vi "GeolocationEnergySNRvariationTxswitching.vi"() -> ()   [LabVIEW 2012]
uses:
  <vilib>/addons/database/Connection.llb/DB Tools Open Connec (Path).vi
  <vilib>/measure/maspectr.llb/FFT Power Spectrum and PSD for 1 Chan.vi
  <instrlib>/niUSRP/niUSRP Fetch Rx Data (CDB Cluster).vi
  <vilib>/addons/Modulation/Digital/General/MT Generate PSK System Parameters(M).vi
  <instrlib>/niUSRP/niUSRP Write Tx Data (CDB Cluster).vi
  <vilib>/addons/Modulation/niDMT.lvlib
  <vilib>/measure/NI_MAPro.lvlib
  <vilib>/addons/database/NI_Database_API.lvlib
panel:
  out "Power Spectrum / PSD":cluster{"f0":dbl, "df":dbl, "magnitude":dbl[]} {"magnitude" format="%.2p"; "f0" format="%0.2p"; "df" format="%0.2p"}
  out "SNR":dbl
  out "x/y":dbl
  in  "IQ rate":dbl=100000.0 format="%#_6p"
  in  "gain":dbl format="%#_6f"
  out "Channel is free":bool
  in  "Boolean":bool
  out "data":variant[][](array[variant])
  out "columns":string[](array[string])
  in  "connection information":path
  out "product":i32
  out "output array":variant[](array[variant])
  out "cluster":T1
  out "data 2":dbl
  out "String":string
  out "millisecond timer value":u32
  out "Entering into 2nd \n          Loop":string
  out "Symbol Rate\n[symbols/sec]":dbl=25000.0 format="%#.6p"
  in  "BPSK System Parameters 9":T2={"Samples per Symbol"=8, "symbol map"=[], "Differential PSK"=enum."disable", "PSK type"=0} caption="BPSK System Parameters" {"PSK type" items=["normal", "shifted", "offset"]; "symbol map" format="%.3f"}
  in  "BPSK System Parameters 8":T2={"Samples per Symbol"=8, "symbol map"=[], "Differential PSK"=enum."disable", "PSK type"=0} caption="BPSK System Parameters" {"PSK type" items=["normal", "shifted", "offset"]; "symbol map" format="%.3f"}
  in  "BPSK System Parameters 7":T2={"Samples per Symbol"=8, "symbol map"=[], "Differential PSK"=enum."disable", "PSK type"=0} caption="BPSK System Parameters" {"PSK type" items=["normal", "shifted", "offset"]; "symbol map" format="%.3f"}
  in  "BPSK System Parameters 6":T2={"Samples per Symbol"=8, "symbol map"=[], "Differential PSK"=enum."disable", "PSK type"=0} caption="BPSK System Parameters" {"PSK type" items=["normal", "shifted", "offset"]; "symbol map" format="%.3f"}
  in  "BPSK System Parameters 5":T2={"Samples per Symbol"=8, "symbol map"=[], "Differential PSK"=enum."disable", "PSK type"=0} caption="BPSK System Parameters" {"PSK type" items=["normal", "shifted", "offset"]; "symbol map" format="%.3f"}
  in  "BPSK System Parameters 4":T2={"Samples per Symbol"=8, "symbol map"=[], "Differential PSK"=enum."disable", "PSK type"=0} caption="BPSK System Parameters" {"PSK type" items=["normal", "shifted", "offset"]; "symbol map" format="%.3f"}
  in  "BPSK System Parameters 3":T2={"Samples per Symbol"=8, "symbol map"=[], "Differential PSK"=enum."disable", "PSK type"=0} caption="BPSK System Parameters" {"PSK type" items=["normal", "shifted", "offset"]; "symbol map" format="%.3f"}
  in  "Tab Control":T3(tab)
  in  "Enter control signal (1,2 or 3)":string
  in  "Packet Parameters":T4={"Guard Bits "=30, "Sync Bits"=20, "Message Bits"=128}
  in  "Packet Pad \n[samples]":i32=200
  in  "Blank Frame \n[samples]":i32=500
  out "Number of Packets in Message":i32=46
  in  "PN sequence order\nfor Sync Bits":i32=31 caption="PN sequence order (9)"
  in  "Packet Repeat":i32=2
  in  "Pulse Shaping Filter Parameters":T5={"Alpha"=0.5, "Filter Length"=6, "TX Filter"=enum."Root Raised Cos"} caption="Pulse Shaping Filter" {"Alpha" format="%.2f"}
  out "Actual Tx Parameters":T6={"Tx IQ Sampling\nRate [s/sec]"=200000.0, "Tx Frequency [Hz]"=2500000000.0, "Tx Gain [dB]"=0.0, "Tx Antenna"="TX1"} {"Tx Gain [dB]" format="%#.6p"; "Tx Frequency [Hz]" format="%#.6p"; "Tx IQ Sampling\nRate [s/sec]" format="%#.6p"}
  in  "USRP IP address":refnum<k15>="192.168.10.2"
  out "error out":errorcluster
  in  "Queue Length":i32=10
  out "Transmission\n       Stop":bool
  in  "end of data?":bool
  out "Constellation Graph":T7(graph)
  in  "autoscale":bool
  out "millisecond timer value 2":u32
  out "x = y?":bool
  out "Transmission\n      Time":bool
  out "error out 2":errorcluster
  out "Message Text 3":string="Two roads diverged in a yellow wood,\nAnd sorry I could not travel both\nAnd be one traveler, long I stood\nAnd looked down one as far as I could\nTo where it bent in the undergrowth.\n\nThen took the other, as just as fair,\nAnd having perhaps the better claim,\nBecause it was grassy and wanted wear;\nThough as for that the passing there\nHad worn them really about the same.\n\nAnd both that morning equally lay\nIn leaves no step had trodden black.\nOh, I kept the first for another day!\nYet knowing how way leads on to way,\nI doubted if I should ever come back.\n\nI shall be telling this with a sigh\nSomewhere ages and ages hence:\nTwo roads diverged in a wood, and I--\nI took the one less traveled by,\nAnd that has made all the difference.\n"
  out "M-PSK (4)":i32
  out "Required Power":dbl
  in  "Referance Cluster":T6={"Tx IQ Sampling\nRate [s/sec]"=500000.0, "Tx Frequency [Hz]"=2500000000.0, "Tx Gain [dB]"=0.0, "Tx Antenna"="TX1"} {"Tx Gain [dB]" format="%#.6p"; "Tx Frequency [Hz]" format="%#.6p"; "Tx IQ Sampling\nRate [s/sec]" format="%#.6p"}
  out "output cluster":T6
  out "Numeric":u32
  # "Guard\nBand"
  # "Sync\nSeq"
  # "Packet\nNumber"
  # "Pad\nData"
  # "Blank\nFrame"
  # "Data"
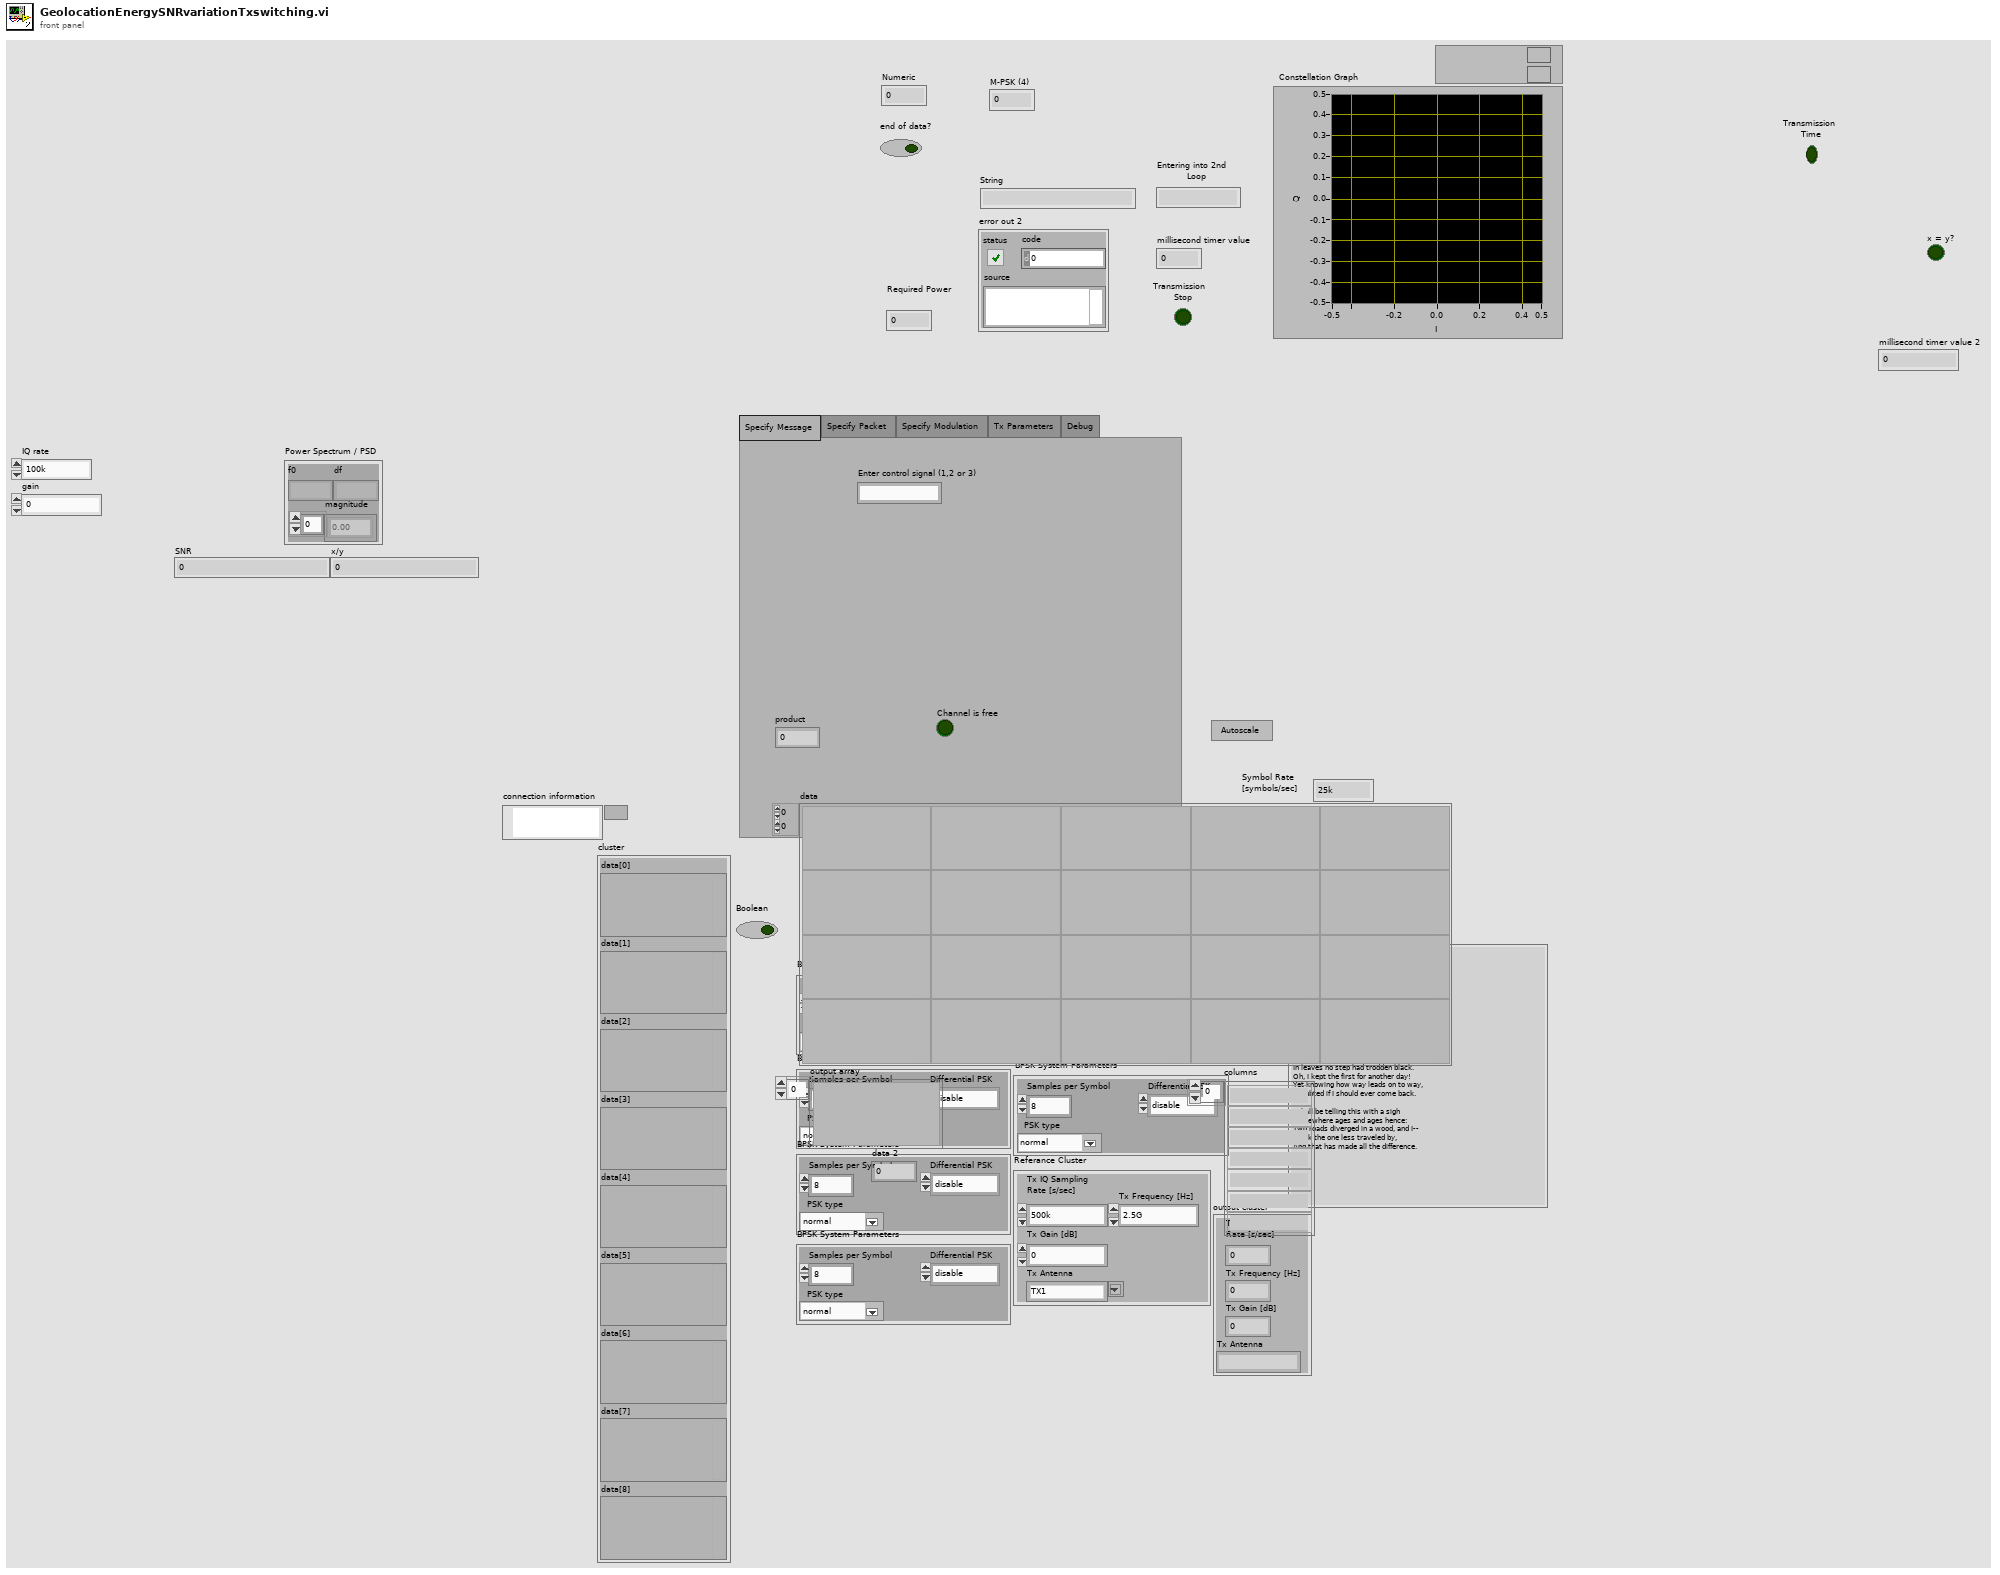
[diagram p1: front panel]
types:
  T1 = cluster{"data[0]":variant, "data[1]":variant, "data[2]":variant, "data[3]":variant, "data[4]":variant, "data[5]":variant, "data[6]":variant, "data[7]":variant, "data[8]":variant}
  T2 = cluster{"Samples per Symbol":i32, "symbol map":cdb[], "Differential PSK":enum16{"disable", "enable"}, "PSK type":u16}
  T3 = enum32{"Specify Message", "Specify Packet", "Specify Modulation", "Tx Parameters", "Debug"}
  T4 = cluster{"Guard Bits ":i32, "Sync Bits":i32, "Message Bits":i32}
  T5 = cluster{"Alpha":dbl, "Filter Length":i32, "TX Filter":enum16{"none", "Raised Cosine", "Root Raised Cos", "Gaussian"}}
  T6 = cluster{"Tx IQ Sampling\nRate [s/sec]":dbl, "Tx Frequency [Hz]":dbl, "Tx Gain [dB]":dbl, "Tx Antenna":string}
  T7 = cluster{"Decimated Array":dbl[], "Decimated Array":dbl[]}[]
  T8 = typedef "NI_Database_API.lvlib/Conn ObjectReference.ctl" = refnum<k1>
  T9 = cluster{"samples per symbol (16)":i32, "symbol map":cdb[], "differential PSK":enum16{"disable", "enable"}, "PSK type":u16}
  T10 = cluster{"s? t:f":cluster{"t0":dbl, "dt":dbl, "Y":cdb[]}, i32}
  T11 = cluster{"output complex waveform":cluster{"t0":dbl, "dt":dbl, "Y":cdb[]}, i32}
  T12 = cluster{"constellation":dbl[], "oversampled data":dbl[]}[]
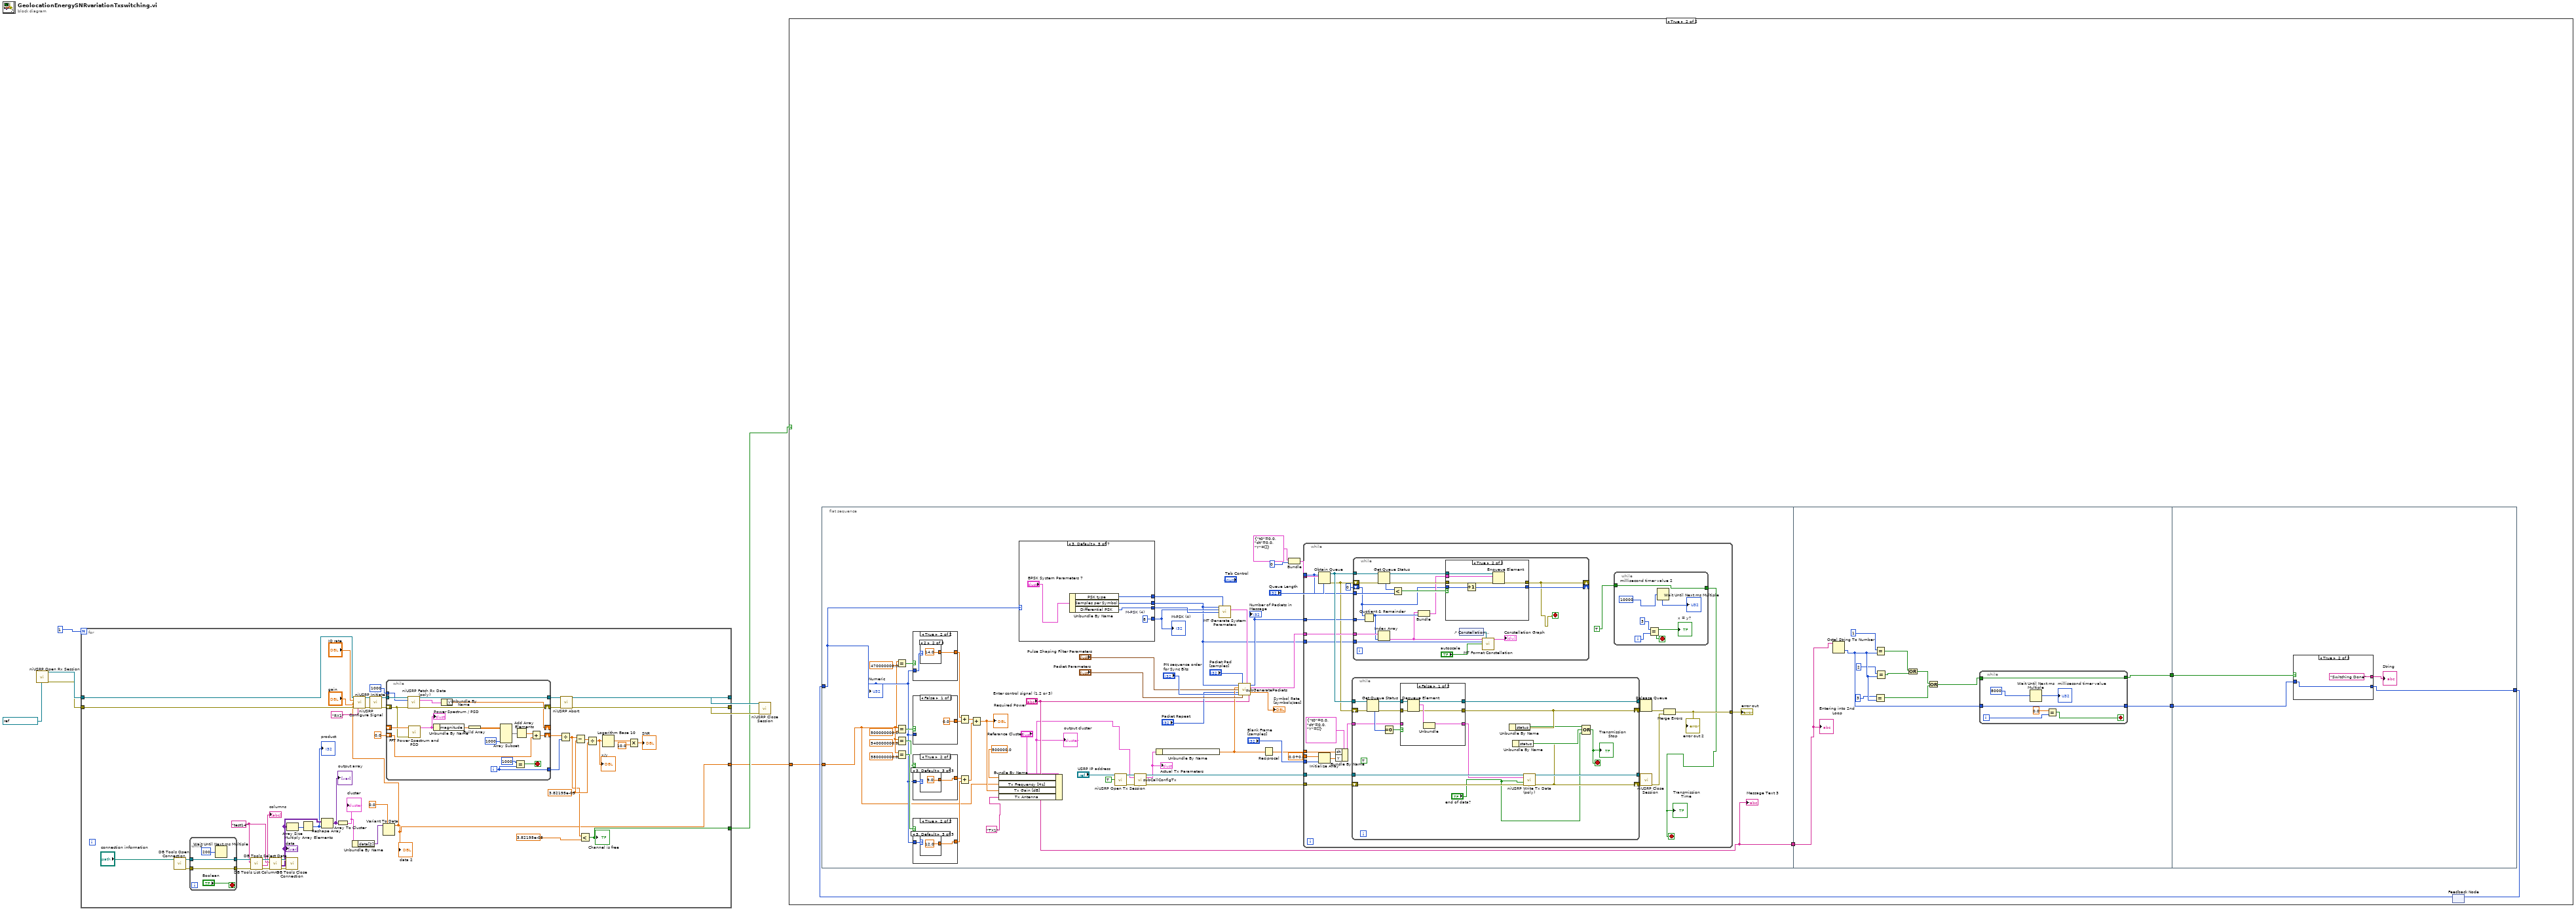
[diagram p0: block diagram]
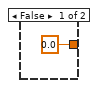
[diagram p3: hidden frame]
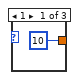
[diagram p4: hidden frame]
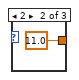
[diagram p5: hidden frame]
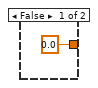
[diagram p6: hidden frame]
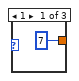
[diagram p7: hidden frame]
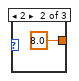
[diagram p8: hidden frame]
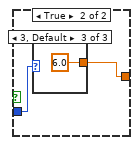
[diagram p9: hidden frame]
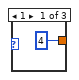
[diagram p10: hidden frame]
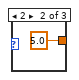
[diagram p11: hidden frame]
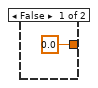
[diagram p12: hidden frame]
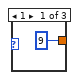
[diagram p13: hidden frame]
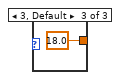
[diagram p14: hidden frame]
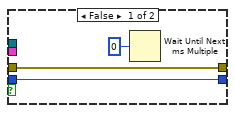
[diagram p15: hidden frame]
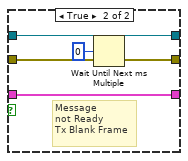
[diagram p16: hidden frame]
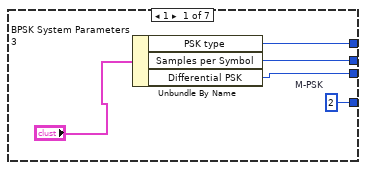
[diagram p17: hidden frame]
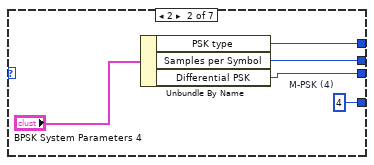
[diagram p18: hidden frame]
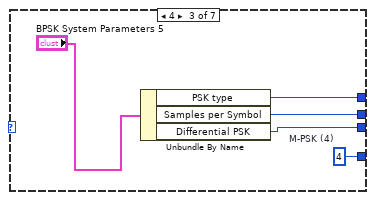
[diagram p19: hidden frame]
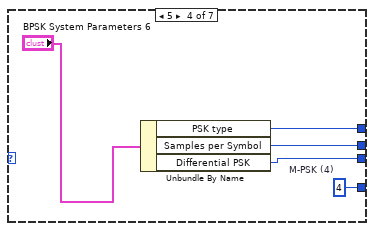
[diagram p20: hidden frame]
diagram:
  n1 = call <instrlib>:"niUSRP Open Rx Session.vi"("device names"=refnum<k15> "192.168.10.4") -> ("session handle out"=w8:refnum<k15>, "error out"=w7:errorcluster)  [unwired: 13 in]
  n2 = for {
    N: 1 -> [_]
    tunnel: w8 -> [w53]
    tunnel: w7 -> [w50]
    tunnel: [w36] -> w4
    tunnel: [w35] -> w3
    tunnel: [w10] -> w2
    tunnel: [w9] -> w1
    w20 = "test14" ("table")
    w32 = 3.82195e-05 ("y")
    n3 = call-poly <vilib>:"DB Tools Open Connection.vi"("connection information"="connection information") -> ("error out"=w24:errorcluster, "connection reference"=w28:T8)  [unwired: 7 in]
    n4 = while {
      tunnel: w28 -> [w55]
      tunnel: [w55] -> w27
      tunnel: w24 -> [w54]
      tunnel: [w54] -> w23
      stop <- "Boolean" stop-if-true
      n5 = Wait Until Next ms Multiple(millisecond multiple=u32 200) -> ()  [unwired: 1 out]
    }
    n6 = call <vilib>:"DB Tools List Columns.vi"("error in (no error)"=w23, "table"=w20, "connection reference"=w27) -> ("error out"=w22:errorcluster, "columns"=→"columns":string[], "connection reference out"=w26:T8)  [unwired: 1 in, 1 out]
    n7 = call <vilib>:"DB Tools Select Data.vi"("error in (no error)"=w22, "table"=w20, "connection reference"=w26) -> ("error out"=w21:errorcluster, "data"=w16:variant[][], "connection reference out"=w25:T8)  [unwired: 3 in]
    "data" <- w16
    n8 = call <vilib>:"DB Tools Close Connection.vi"("error in (no error)"=w21, "connection reference"=w25) -> ()  [unwired: 5 in, 1 out]
    n9 = Array Size(array=w16) -> (size(s)=w17:i32[])
    n10 = Multiply Array Elements(1:w17) -> (0:w15:i32)
    "product" <- w15
    n11 = Reshape Array(w16, w15) -> (w14:variant[])
    "output array" <- w14
    n12 = Array To Cluster(array=w14) -> (cluster=w13:T1)
    "cluster" <- w13
    n13 = Unbundle By Name(w13) -> ("data[2]"=w12:variant)
    n14 = Variant To Data(type=0.0, Variant=w12) -> (data=w9:dbl)  [unwired: 1 in, 1 out]
    "data 2" <- w9
    n15 = call <instrlib>:"niUSRP Configure Signal.vi"("session handle"=w53, "IQ rate"="IQ rate", "carrier frequency"=w9, "gain"="gain", "error in (no error)"=w50, "active antenna"="RX1") -> ("session handle out"=w52:refnum<k15>, "error out"=w51:errorcluster)  [unwired: 5 in, 3 out]
    n16 = call <instrlib>:"niUSRP Initiate.vi"("session handle"=w52, "error in (no error)"=w51) -> ("session handle out"=w49:refnum<k15>, "error out"=w48:errorcluster)  [unwired: 12 in]
    n17 = while {
      tunnel: w49 -> [w76]
      shift-right: [w60] -> w47
      shift-left: w48 -> [w73]
      tunnel: [w75] -> w46
      shift-right: [w58] -> _
      shift-left: _ -> [w74]
      shift-right: [w67] -> w44
      shift-left: 0.0 -> [w68]
      tunnel: [w62] -> w43
      tunnel: 1000 -> [w65]
      i -> [w62]
      stop <- w61 stop-if-true
      n18 = call-poly <instrlib>:"niUSRP Fetch Rx Data (poly).vi"("session handle"=w76, "number of samples"=w65, "error in (no error)"=w73) -> ("session handle out"=w75:refnum<k15>, "data"=w59:cluster{"t0":dbl, "dt":dbl, "Y":cdb[]}, "error out"=w60:errorcluster)  [unwired: 9 in, 1 out]
      n19 = call-poly <vilib>:"FFT Power Spectrum and PSD.vi"("error in (no error)"=w73, "time signal"=w74) -> ("Power Spectrum / PSD"=w72:cluster{"f0":dbl, "df":dbl, "magnitude":dbl[]})  [unwired: 6 in, 3 out]
      "Power Spectrum / PSD" <- w72
      n20 = Unbundle By Name(w72) -> ("magnitude"=w71:dbl[])
      n21 = Unbundle By Name(w59) -> ("Y"=w58:cdb[])
      n22 = Build Array(w71) -> (w70:dbl[][])
      n23 = Array Subset(array=w70, length (col)=1000 ("length")) -> (w69:dbl[][])  [unwired: 3 in]
      n24 = Equal?(x=1000, y=w62) -> (x = y?=w61:bool)
      n25 = Add Array Elements(numeric array=w69) -> (sum=w66:dbl)
      n26 = Add(x=w66, y=w68) -> (x+y=w67:dbl)
    }
    n27 = Divide(x=w44, y=w43) -> (x/y=w30:dbl)
    n28 = call <instrlib>:"niUSRP Abort.vi"("session handle"=w46, "error in (no error)"=w47) -> ("session handle out"=w36:refnum<k15>, "error out"=w35:errorcluster)  [unwired: 12 in]
    n29 = Subtract(x=w30, y=w32) -> (x-y=w31:dbl)
    n30 = Less?(x=w30, y=3.82195e-05) -> (x < y?=w10:bool)
    "Channel is free" <- w10
    n31 = Divide(x=w31, y=w32) -> (x/y=w42:dbl)
    "x/y" <- w42
    n32 = Logarithm Base 10(1:w42) -> (0:w41:dbl)
    n33 = Multiply(x=w41, y=10.0) -> (x*y=→"SNR":dbl)
  }
  n34 = call <instrlib>:"niUSRP Close Session.vi"("session handle"=w4, "error in (no error)"=w3) -> ()  [unwired: 13 in, 1 out]
  n35 = case shown="True" w2 {
    tunnel: w1 -> [_ w77]
    frame False {
    }
    frame True {
      n36 = flat-sequence {
        tunnel: ["Enter control signal (1,2 or 3)"] -> w82
        tunnel: w78 -> [w84]
        tunnel: w77 -> [w83]
        tunnel: w82 -> [w280]
        tunnel: [w282] -> w81
        tunnel: [w281] -> w80
        tunnel: w81 -> [w301]
        tunnel: w80 -> [w300]
        tunnel: [w299] -> w79
        frame #0 {
          n37 = Equal?(x=w83, y=470000000.0) -> (x = y?=w90:bool)
          n38 = Equal?(x=w83, y=500000000.0) -> (x = y?=w91:bool)
          n39 = Equal?(x=w83, y=540000000.0) -> (x = y?=w92:bool)
          n40 = Equal?(x=w83, y=580000000.0) -> (x = y?=w93:bool)
          n41 = case shown="True" w90 {
            tunnel: [0.0 w153] -> w101
            tunnel: w84 -> [_ w154]
            frame False {
            }
            frame True {
              n42 = case shown="2" w154 {
                tunnel: [9 14.0 18.0] -> w153
                frame 1 {
                }
                frame 2 {
                }
                frame 3, Default {
                }
              }
            }
          }
          n43 = case shown="False" w91 {
            tunnel: [0.0 w147] -> w100
            tunnel: w84 -> [_ w148]
            frame False {
            }
            frame True {
              n44 = case shown="3, Default" w148 {
                tunnel: [4 5.0 6.0] -> w147
                frame 1 {
                }
                frame 2 {
                }
                frame 3, Default {
                }
              }
            }
          }
          n45 = case shown="True" w92 {
            tunnel: [0.0 w141] -> w99
            tunnel: w84 -> [_ w142]
            frame False {
            }
            frame True {
              n46 = case shown="3, Default" w142 {
                tunnel: [7 8.0 9.0] -> w141
                frame 1 {
                }
                frame 2 {
                }
                frame 3, Default {
                }
              }
            }
          }
          n47 = case shown="True" w93 {
            tunnel: [0.0 w135] -> w98
            tunnel: w84 -> [_ w136]
            frame False {
            }
            frame True {
              n48 = case shown="3, Default" w136 {
                tunnel: [10 11.0 12.0] -> w135
                frame 1 {
                }
                frame 2 {
                }
                frame 3, Default {
                }
              }
            }
          }
          n49 = Add(x=w101, y=w100) -> (x+y=w103:dbl)
          n50 = Add(x=w99, y=w98) -> (x+y=w102:dbl)
          n51 = Add(x=w103, y=w102) -> (x+y=w88:dbl)
          "Required Power" <- w88
          n52 = Bundle By Name(cluster="Referance Cluster", "Tx IQ Sampling\nRate [s/sec]"=500000.0, "Tx Frequency [Hz]"=w83, "Tx Gain [dB]"=w88, "Tx Antenna"="TX1") -> (w86:T6)
          "output cluster" <- w86
          n53 = case shown="3, Default" w84 {
            tunnel: [w246 w251 w258 w263 w268 w274 w277] -> w107
            tunnel: [w247 w252 w257 w262 w267 w273 w278] -> w133
            tunnel: [w249 w254 w259 w264 w266 w272 0 ("M-PSK (4)")] -> w124
            tunnel: [w248 w253 w256 w261 w269 w271 w279] -> w113
            frame 1 {
              w249 = 2  # M-PSK
              n54 = Unbundle By Name("BPSK System Parameters 3") -> ("PSK type"=w248:u16, "Samples per Symbol"=w246:i32, "Differential PSK"=w247:enum16{"disable", "enable"})
            }
            frame 2 {
              w254 = 4  # M-PSK (4)
              n55 = Unbundle By Name("BPSK System Parameters 4") -> ("PSK type"=w253:u16, "Samples per Symbol"=w251:i32, "Differential PSK"=w252:enum16{"disable", "enable"})
            }
            frame 4 {
              w259 = 4  # M-PSK (4)
              n56 = Unbundle By Name("BPSK System Parameters 5") -> ("PSK type"=w256:u16, "Samples per Symbol"=w258:i32, "Differential PSK"=w257:enum16{"disable", "enable"})
            }
            frame 5 {
              w264 = 4  # M-PSK (4)
              n57 = Unbundle By Name("BPSK System Parameters 6") -> ("PSK type"=w261:u16, "Samples per Symbol"=w263:i32, "Differential PSK"=w262:enum16{"disable", "enable"})
            }
            frame 3, Default {
              w266 = 8  # M-PSK (4)
              n58 = Unbundle By Name("BPSK System Parameters 7") -> ("PSK type"=w269:u16, "Samples per Symbol"=w268:i32, "Differential PSK"=w267:enum16{"disable", "enable"})
            }
            frame 6 {
              w272 = 16  # M-PSK (4)
              n59 = Unbundle By Name("BPSK System Parameters 8") -> ("PSK type"=w271:u16, "Samples per Symbol"=w274:i32, "Differential PSK"=w273:enum16{"disable", "enable"})
            }
            frame 7 {
              n60 = Unbundle By Name("BPSK System Parameters 9") -> ("PSK type"=w279:u16, "Samples per Symbol"=w277:i32, "Differential PSK"=w278:enum16{"disable", "enable"})
            }
          }
          "M-PSK (4)" <- w124
          n61 = call <instrlib>:"niUSRP Open Tx Session.vi"("device names"="USRP IP address", "reset"=TRUE) -> ("session handle out"=w117:refnum<k15>, "error out"=w116:errorcluster)  [unwired: 12 in]
          n62 = call "subCallConfigTx.vi"("session handle"=w117, "Tx Parameters"=w86, "error in"=w116) -> ("session handle out"=w123:refnum<k15>, "Actual Tx Parameters"=w122:T6, "error out"=w126:errorcluster)  [unwired: 10 in]
          "Actual Tx Parameters" <- w122
          n63 = Unbundle By Name(w122) -> ("Tx IQ Sampling\nRate [s/sec]"=w108:dbl)
          n64 = call-poly <vilib>:"MT Generate System Parameters.vi"("samples per symbol (16)"=w107, "PSK type"=w113, "M-PSK (4)"=w124, "differential PSK"=w133) -> ("PSK system parameters"=w114:T9)  [unwired: 9 in, 2 out]
          n65 = call "subGeneratePackets.vi"("Samples per Symbol"=w107, "Packet Pad \n[samples]"="Packet Pad \n[samples]", "PSK system parameters"=w114, "Tx IQ Sampling\nRate [s/sec]"=w108, "Pulse Shaping Filter Parameters"="Pulse Shaping Filter Parameters", "Packet Repeat"="Packet Repeat", "PN sequence order\nfor Sync Bits"="PN sequence order\nfor Sync Bits", "Packet Parameters"="Packet Parameters", "Message Text"="Enter control signal (1,2 or 3)") -> ("Number of Packets"=w121:i32, "Packets"=w127:cluster{"t0":dbl, "dt":dbl, "Y":cdb[]}[], "Symbol Rate"=→"Symbol Rate\n[symbols/sec]":dbl)  [unwired: 4 in]
          "Number of Packets in Message" <- w121
          n66 = Reciprocal(x=w108) -> (1/x=w125:dbl)
          n67 = Bundle("s? t:f"=cluster{"t0":dbl, "dt":dbl, "Y":cdb[]} {"t0"=0.0, "dt"=0.0, "Y"=[]}, 0) -> (w129:T10)  [unwired: 1 in]
          n68 = while {
            tunnel: cdb 0.0+0.0i ("element") -> [w182]
            tunnel: "Blank Frame \n[samples]" -> [w181]
            tunnel: w129 -> [w175]
            tunnel: "Queue Length" -> [w173]
            tunnel: w127 -> [w172]
            tunnel: w126 -> [w171]
            tunnel: w125 -> [w168]
            tunnel: w123 -> [w167]
            tunnel: w121 -> [w166]
            tunnel: [w161] -> w112
            tunnel: w107 -> [w160]
            stop <- w158 stop-if-true
            n69 = Obtain Queue(max queue size (-1, unlimited)=w173, element data type=w175) -> (queue out=w180:refnum<queue>, error out=w164:errorcluster)  [unwired: 3 in, 1 out]
            n70 = Initialize Array(w182, w181) -> (w179:cdb[])
            n71 = Bundle By Name(cluster=cluster{"t0":dbl, "dt":dbl, "Y":cdb[]} {"t0"=0.0, "dt"=0.0, "Y"=[]} ("s? t:f"), "dt"=w168, "Y"=w179) -> (w178:cluster{"t0":dbl, "dt":dbl, "Y":cdb[]})
            n72 = while {
              tunnel: w167 -> [w225]
              shift-right: [w222] -> w170
              shift-left: w171 -> [w226]
              tunnel: w180 -> [w234]
              tunnel: w178 -> [w231]
              tunnel: [w230] -> w177
              tunnel: [w224] -> w169
              shift-right: [w221] -> w176
              shift-left: w164 -> [w227]
              stop <- w218 stop-if-true
              (unwired) TRUE
              n73 = Get Queue Status(queue=w234, error in (no error)=w227) -> (queue out=w229:refnum<queue>, error out=w228:errorcluster, # elements in queue=w233:i32)  [unwired: 1 in, 5 out]
              n74 = Equal To 0?(x=w233) -> (x = 0?=w232:bool)
              n75 = case shown="False" w232 {
                tunnel: w231 -> [_ w244]
                tunnel: [w236 w244] -> w219
                tunnel: [w240 w242] -> w230
                tunnel: [w235 w243] -> w221
                tunnel: w229 -> [w239 w242]
                tunnel: w228 -> [w238 w243]
                frame False {
                  n76 = Dequeue Element(queue=w239, error in (no error)=w238) -> (queue out=w240:refnum<queue>, element=w237:T10, error out=w235:errorcluster)  [unwired: 1 in, 1 out]
                  n77 = Unbundle(w237) -> ("s? t:f"=w236:cluster{"t0":dbl, "dt":dbl, "Y":cdb[]})  [unwired: 1 out]
                }
                frame True {
                  # "Message\nnot Ready\nTx Blank Frame"
                  n78 = Wait Until Next ms Multiple(millisecond multiple=u32 0) -> ()  [unwired: 1 out]
                }
              }
              n79 = Unbundle By Name(w221) -> ("status"=w220:bool)
              n80 = call-poly <instrlib>:"niUSRP Write Tx Data (poly).vi"("session handle"=w225, "data"=w219, "end of data?"="end of data?", "error in (no error)"=w226) -> ("session handle out"=w224:refnum<k15>, "error out"=w222:errorcluster)  [unwired: 10 in]
              n81 = Unbundle By Name(w222) -> ("status"=w223:bool)
              n82 = Compound Arithmetic op=OR(w220, w223, "end of data?") -> (w218:bool)
              "Transmission\n       Stop" <- w218
            }
            n83 = while {
              tunnel: w180 -> [w207]
              shift-right: [w200] -> _
              shift-left: 0 -> [w196]
              tunnel: w172 -> [w197]
              tunnel: w173 -> [w199]
              tunnel: w166 -> [w198]
              shift-right: [w189] -> _
              shift-left: w164 -> [w202]
              tunnel: w160 -> [w192]
              stop <- w189 stop-if-true
              n84 = Quotient & Remainder(x=w196, y=w198) -> (x-y*floor(x/y)=w195:i32)  [unwired: 1 out]
              n85 = Index Array(array=w197, index=w195) -> (element=w190:cluster{"t0":dbl, "dt":dbl, "Y":cdb[]})
              n86 = Get Queue Status(queue=w207, error in (no error)=w202) -> (queue out=w206:refnum<queue>, error out=w203:errorcluster, # elements in queue=w205:i32)  [unwired: 1 in, 5 out]
              n87 = Less?(x=w205, y=w199) -> (x < y?=w204:bool)
              n88 = Bundle("output complex waveform"=w190, w195) -> (w201:T11)  [unwired: 1 in]
              n89 = case shown="True" w204 {
                tunnel: w203 -> [w208 w216]
                tunnel: w206 -> [_ w215]
                tunnel: [w208 w214] -> w189
                tunnel: w201 -> [_ w213]
                tunnel: w196 -> [w210 w212]
                tunnel: [w210 w211] -> w200
                frame False {
                  n90 = Wait Until Next ms Multiple(millisecond multiple=u32 0) -> ()  [unwired: 1 out]
                }
                frame True {
                  n91 = Increment(x=w212) -> (x+1=w211:i32)
                  n92 = Enqueue Element(queue=w215, element=w213, error in (no error)=w216) -> (error out=w214:errorcluster)  [unwired: 1 in, 2 out]
                }
              }
              n93 = control-ref of="Constellation Graph"() -> (w193:refnum<vi>)
              n94 = call <vilib>:"MT Format Constellation.vi"("waveform"=w190, "constellation reference"=w193, "samples per symbol"=w192, "autoscale"="autoscale") -> ("constellation graph"=→"Constellation Graph":T12)  [unwired: 1 in, 10 out]
            }
            n95 = while {
              tunnel: TRUE -> [w188]
              tunnel: [w188] -> w158
              i -> [w186]
              stop <- w185 stop-if-true
              n96 = Equal?(x=3, y=w186) -> (x = y?=w185:bool)
              "x = y?" <- w185
              n97 = Wait Until Next ms Multiple(millisecond multiple=u32 10000) -> (millisecond timer value=→"millisecond timer value 2":u32)
            }
            "Transmission\n      Time" <- w158
            n98 = Release Queue(queue=w177, error in (no error)=w176) -> (error out=w163:errorcluster)  [unwired: 3 out]
            n99 = call <instrlib>:"niUSRP Close Session.vi"("session handle"=w169, "error in (no error)"=w170) -> ("error out"=w162:errorcluster)  [unwired: 13 in]
            n100 = Merge Errors(w163, w162) -> (w161:errorcluster)
            "error out 2" <- w161
          }
          "error out" <- w112
          "Message Text 3" <- "Enter control signal (1,2 or 3)"
          "Numeric" <- w84
        }
        frame #1 {
          n101 = Octal String To Number(4:w280) -> (0:w286:u32)  [unwired: 2 in, 1 out]
          n102 = Equal?(x=3, y=w286) -> (x = y?=w288:bool)
          n103 = Equal?(x=1, y=w286) -> (x = y?=w291:bool)
          n104 = Equal?(x=2, y=w286) -> (x = y?=w290:bool)
          n105 = Or(x=w291, y=w290) -> (x .or. y?=w289:bool)
          n106 = Or(x=w289, y=w288) -> (x .or. y?=w287:bool)
          n107 = while {
            tunnel: w287 -> [w297]
            tunnel: [w297] -> w282
            tunnel: w286 -> [w296]
            tunnel: [w296] -> w281
            i -> [w294]
            stop <- w293 stop-if-true
            n108 = Wait Until Next ms Multiple(millisecond multiple=u32 8000) -> (millisecond timer value=→"millisecond timer value":u32)
            n109 = Equal?(x=0.0, y=w294) -> (x = y?=w293:bool)
          }
          "Entering into 2nd \n          Loop" <- w280
        }
        frame #2 {
          n110 = case shown="True" w301 {
            tunnel: ["Not Done" "Switching Done"] -> w302
            tunnel: [_ w304] -> w299
            tunnel: w300 -> [_ w304]
            frame False {
            }
            frame True {
            }
          }
          "String" <- w302
        }
      }
      n111 = feedback #1() -> (w78:u32)  [unwired: 1 in]
      n112 = feedback-in #1(w79) -> ()
    }
  }
